vi "scriptEventSCMenuSelection.vi"(8 "error in (no error)":errorcluster, 10 "path":string, 11 "ScriptEditorV2 in":refnum<class "ScriptEditorV2.lvclass">) -> (0 "error out":errorcluster, 3 "ScriptEditorV2 out":refnum<class "ScriptEditorV2.lvclass">)   [LabVIEW 2011, in "Views.lvlib" / "ScriptEditor.lvlib" / "ScriptEditorV2.lvclass"]
uses:
  ScriptEditorV2.lvclass
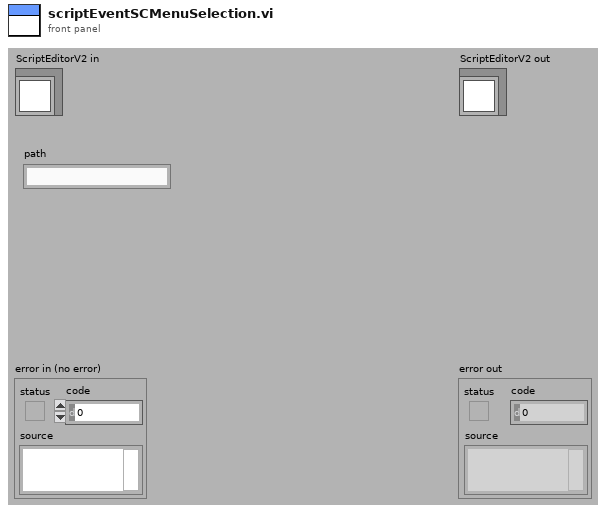
[diagram p1: front panel]
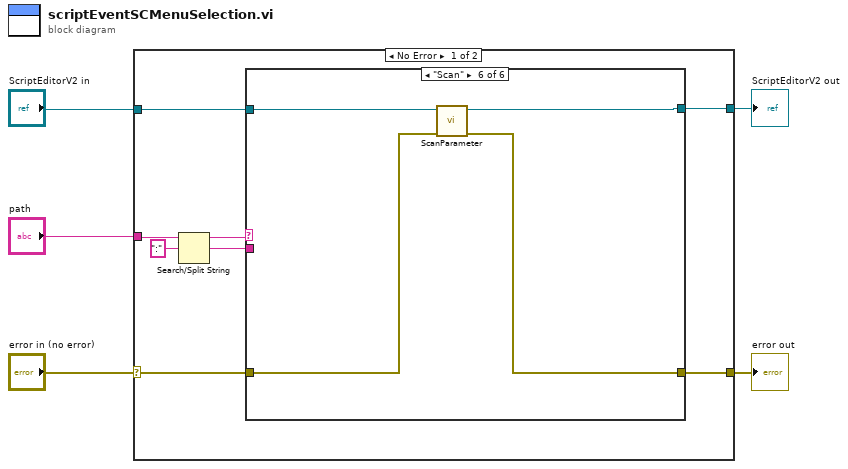
[diagram p0: block diagram]
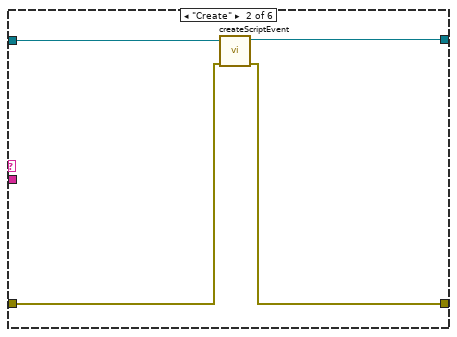
[diagram p3: hidden frame]
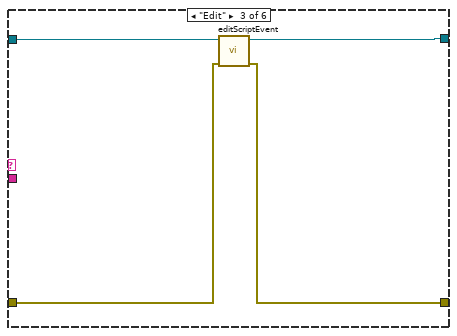
[diagram p4: hidden frame]
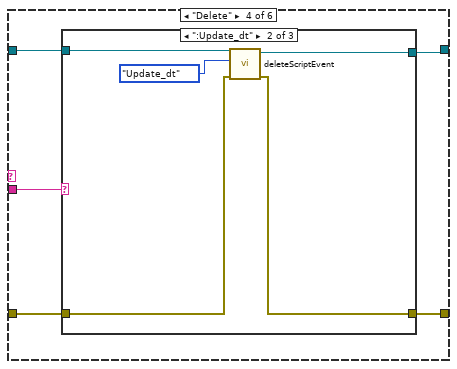
[diagram p5: hidden frame]
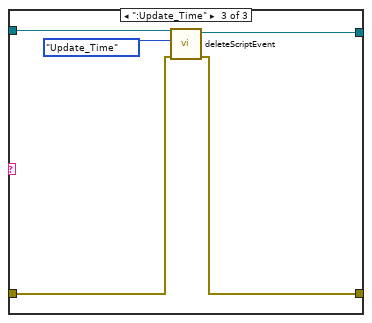
[diagram p7: hidden frame]
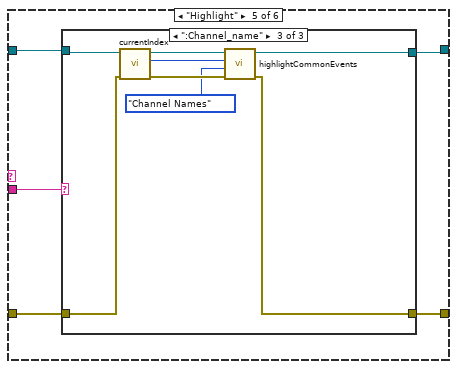
[diagram p8: hidden frame]
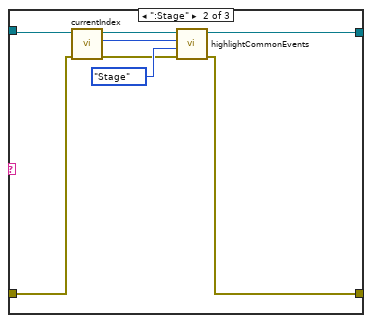
[diagram p10: hidden frame]
diagram:
  n1 = case shown="No Error" "error in (no error)" {
    selector: "error in (no error)" -> [w12 w69]
    tunnel: [w11 w69] -> w2
    tunnel: [w13 w68] -> w4
    tunnel: "path" -> [w10 _]
    tunnel: "ScriptEditorV2 in" -> [w6 w68]
    frame No Error {
      n2 = Search/Split String(string=w10, search string/char (-)=":") -> (substring before match=w8:string, match + rest of string=w7:string)  [unwired: 1 in, 1 out]
      n3 = case shown="\"Scan\"" w8 {
        tunnel: [w14 w19 w22 w24 w41 w66] -> w13
        tunnel: w12 -> [w15 w18 w21 w27 w44 w65]
        tunnel: [w15 w17 w20 w26 w43 w64] -> w11
        tunnel: w7 -> [_ _ _ w28 w45 _]
        tunnel: w6 -> [w14 w16 w23 w25 w42 w67]
        frame Default {
        }
        frame "Create" {
          n4 = call "createScriptEvent.vi"("error in (no error)"=w18, "ScriptEditorV2 in"=w16) -> ("error out"=w17:errorcluster, "ScriptEditorV2 out"=w19:refnum<class "ScriptEditorV2.lvclass">)  [unwired: 8 in]
        }
        frame "Edit" {
          n5 = call "editScriptEvent.vi"("error in (no error)"=w21, "ScriptEditorV2 in"=w23) -> ("error out"=w20:errorcluster, "ScriptEditorV2 out"=w22:refnum<class "ScriptEditorV2.lvclass">)  [unwired: 8 in]
        }
        frame "Delete" {
          n6 = case shown="\":Update_dt\"" w28 {
            tunnel: w27 -> [w30 w33 w38]
            tunnel: [w30 w32 w37] -> w26
            tunnel: w25 -> [w29 w35 w40]
            tunnel: [w29 w31 w39] -> w24
            frame Default {
            }
            frame ":Update_dt" {
              n7 = call "deleteScriptEvent.vi"("error in (no error)"=w33, "Enum"=enum16{"Update_dt", "Update_Time"}."Update_dt", "ScriptEditorV2 in"=w35) -> ("error out"=w32:errorcluster, "ScriptEditorV2 out"=w31:refnum<class "ScriptEditorV2.lvclass">)  [unwired: 7 in]
            }
            frame ":Update_Time" {
              n8 = call "deleteScriptEvent.vi"("error in (no error)"=w38, "Enum"=enum16{"Update_dt", "Update_Time"}."Update_Time", "ScriptEditorV2 in"=w40) -> ("error out"=w37:errorcluster, "ScriptEditorV2 out"=w39:refnum<class "ScriptEditorV2.lvclass">)  [unwired: 7 in]
            }
          }
        }
        frame "Highlight" {
          n9 = case shown="\":Channel_name\"" w45 {
            tunnel: w44 -> [w47 w49 w56]
            tunnel: [w47 w54 w58] -> w43
            tunnel: w42 -> [w46 w52 w61]
            tunnel: [w46 w55 w59] -> w41
            frame Default {
            }
            frame ":Stage" {
              n10 = call "currentIndex.vi"("error in (no error)"=w49, "ScriptEditorV2 in"=w52) -> ("error out"=w48:errorcluster, "index"=w50:i32, "ScriptEditorV2 out"=w51:refnum<class "ScriptEditorV2.lvclass">)  [unwired: 7 in]
              n11 = call "highlightCommonEvents.vi"("error in (no error)"=w48, "Enum"=enum16{"Channel Names", "Stage"}."Stage", "rowIndex"=w50, "ScriptEditorV2 in"=w51) -> ("error out"=w54:errorcluster, "ScriptEditorV2 out"=w55:refnum<class "ScriptEditorV2.lvclass">)  [unwired: 6 in]
            }
            frame ":Channel_name" {
              n12 = call "currentIndex.vi"("error in (no error)"=w56, "ScriptEditorV2 in"=w61) -> ("error out"=w62:errorcluster, "index"=w63:i32, "ScriptEditorV2 out"=w60:refnum<class "ScriptEditorV2.lvclass">)  [unwired: 7 in]
              n13 = call "highlightCommonEvents.vi"("error in (no error)"=w62, "Enum"=enum16{"Channel Names", "Stage"}."Channel Names", "rowIndex"=w63, "ScriptEditorV2 in"=w60) -> ("error out"=w58:errorcluster, "ScriptEditorV2 out"=w59:refnum<class "ScriptEditorV2.lvclass">)  [unwired: 6 in]
            }
          }
        }
        frame "Scan" {
          n14 = call "ScanParameter.vi"("error in (no error)"=w65, "ScriptEditorV2 in"=w67) -> ("error out"=w64:errorcluster, "ScriptEditorV2 out"=w66:refnum<class "ScriptEditorV2.lvclass">)  [unwired: 8 in]
        }
      }
    }
    frame Error {
    }
  }
  "error out" <- w2
  "ScriptEditorV2 out" <- w4
